vi "ChangePassword.vi"(3 "error in (no error)":errorcluster, 5 "连接模式":enum16{"单机", "联网"}(ring)) -> (0 "error out":errorcluster)   [LabVIEW 2017]
uses:
  <vilib>/Utility/error.llb/DialogType.ctl
  <vilib>/addons/database/Connection.llb/DB Tools Open Connec (String).vi
  <vilib>/addons/database/Connection.llb/Conn Execute.vi
  <vilib>/addons/database/Recordset.llb/Rec Destroy - Connection.vi
  <vilib>/addons/database/NI_Database_API.lvlib
panel:
  in  "取消":bool
  in  "确定":bool
  in  "显示密码":bool
  in  "重复新密码":string
  in  "新   密   码":string
  in  "原   密   码":string
  in  "用   户   名":string(combo)
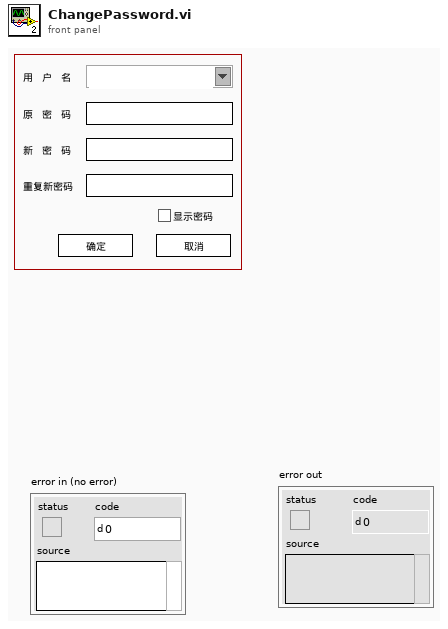
[diagram p1: front panel]
types:
  T1 = typedef "DialogType.ctl" = u16
  T2 = typedef "NI_Database_API.lvlib/Conn ObjectReference.ctl" = refnum<k1>
  T3 = typedef "NI_Database_API.lvlib/Rec ObjectReference.ctl" = refnum<k1>
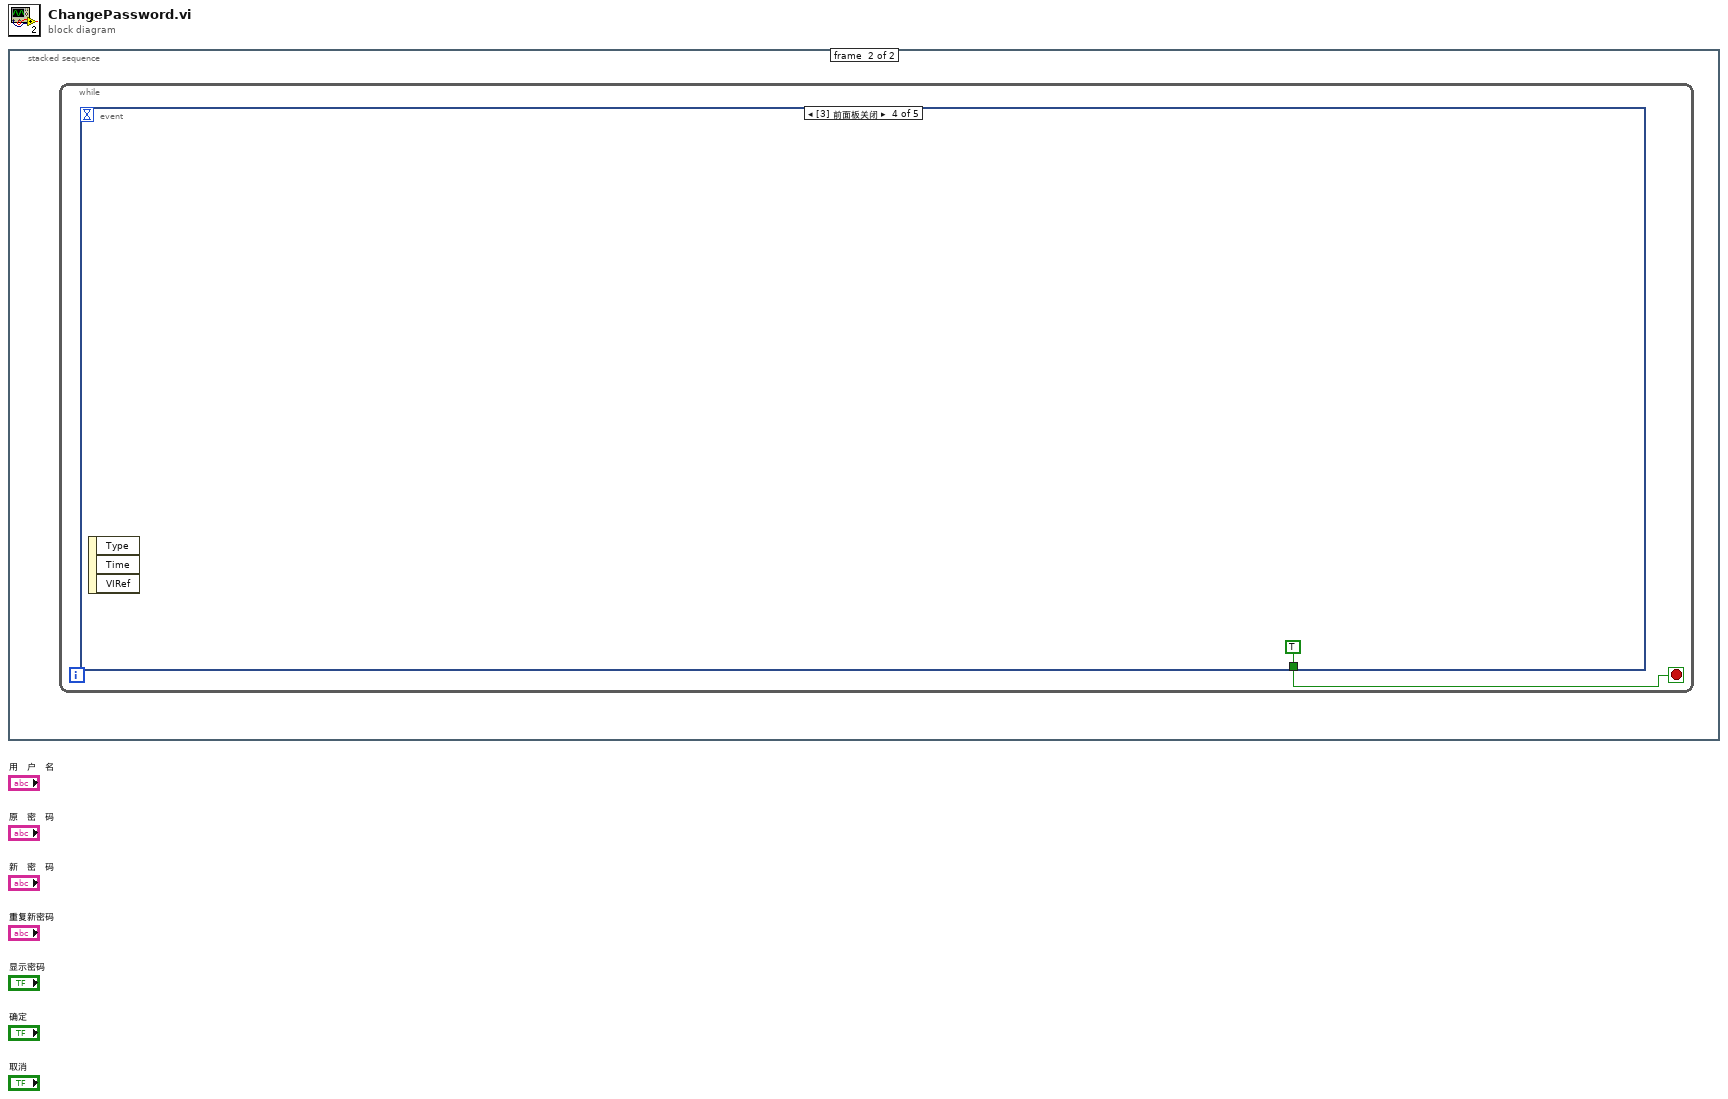
[diagram p0: block diagram]
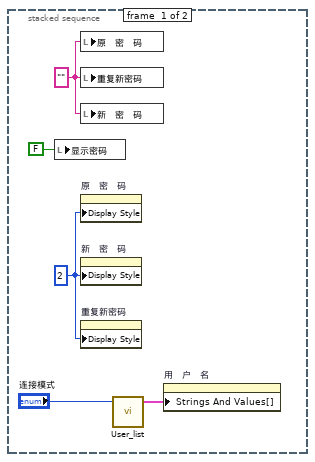
[diagram p2: hidden frame]
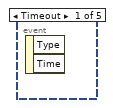
[diagram p3: hidden frame]
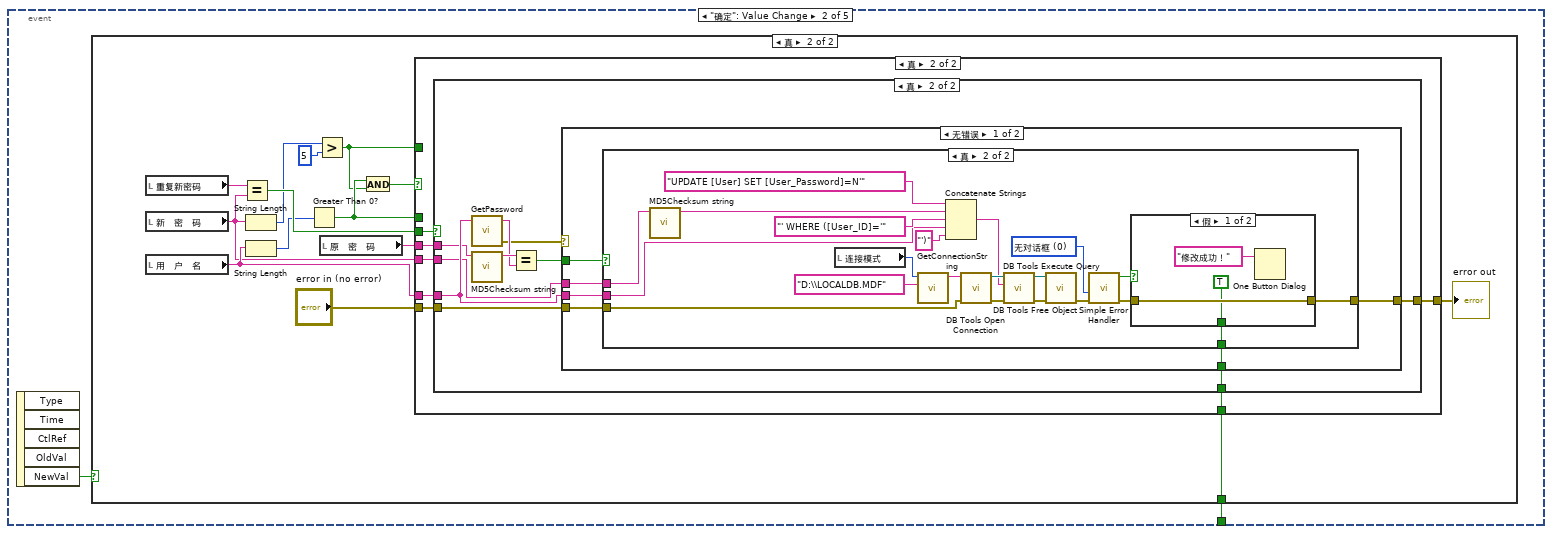
[diagram p4: hidden frame]
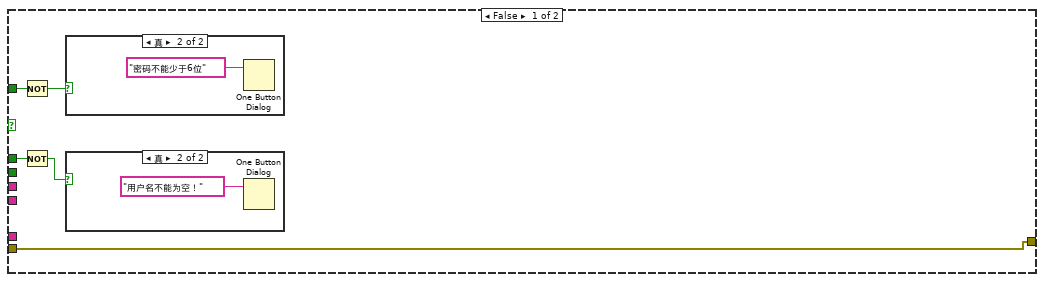
[diagram p6: hidden frame]
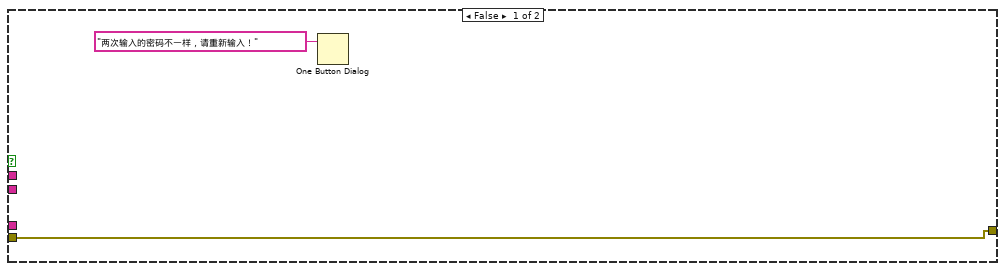
[diagram p9: hidden frame]
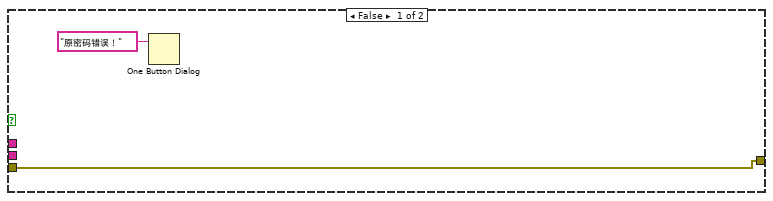
[diagram p10: hidden frame]
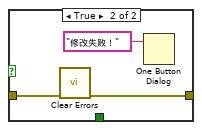
[diagram p11: hidden frame]
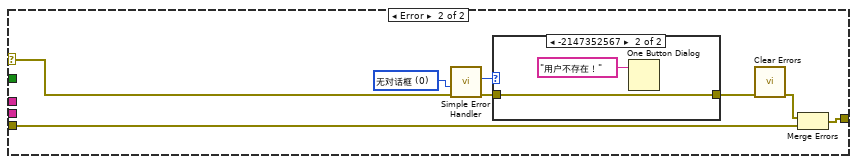
[diagram p12: hidden frame]
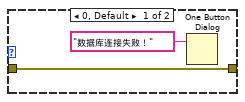
[diagram p13: hidden frame]
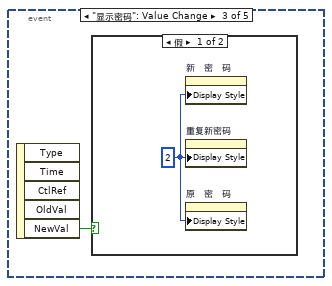
[diagram p14: hidden frame]
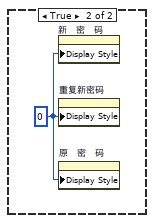
[diagram p15: hidden frame]
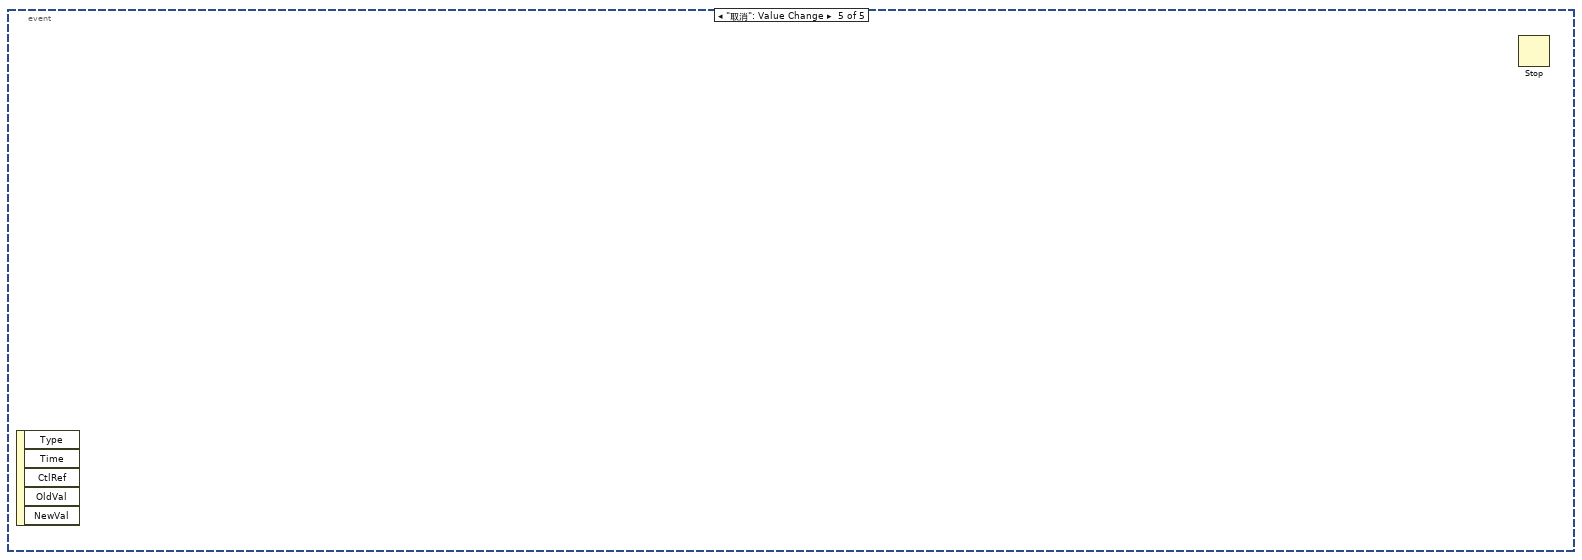
[diagram p16: hidden frame]
diagram:
  n1 = stacked-sequence {
    frame #0 {
      w3 = ""
      w5 = u32 2 ("显示样式")
      n2 = local write "显示密码"(FALSE ("显示密码")) -> ()
      n3 = local write "原   密   码"(w3) -> ()
      n4 = local write "重复新密码"(w3) -> ()
      n5 = local write "新   密   码"(w3) -> ()
      n6 = property on="原   密   码" class="Str"("Display Style"=w5) -> ()  [unwired: 2 in, 2 out]
      n7 = property on="新   密   码" class="Str"("Display Style"=w5) -> ()  [unwired: 2 in, 2 out]
      n8 = property on="重复新密码" class="Str"("Display Style"=w5) -> ()  [unwired: 2 in, 2 out]
      n9 = call "User_list.vi"("连接模式"="连接模式") -> ("User_list"=w2:cluster{string, string}[])  [unwired: 3 in, 1 out]
      n10 = property on="用   户   名" class="CmbBox"("Strings And Values[]"=w2) -> ()  [unwired: 2 in, 2 out]
    }
    frame #1 {
      n11 = while {
        stop <- w6 stop-if-true
        n12 = event shown="[3] 前面板关闭" {
          selector: _ -> [_ _ _ _ _]
          dyn-events: _ -> [_ _ _ _ _]
          timeout: _ -> [_ _ _ _ _]
          tunnel: [_ w7 _ TRUE _] -> w6
          event Timeout {
            n13 = event-data() -> ()  [unwired: 1 in, 2 out]
          }
          event "确定": Value Change {
            n14 = event-data() -> ("NewVal"=w8:bool)  [unwired: 1 in, 4 out]
            n15 = case shown="真" w8 {
              tunnel: [_ w9] -> w7
              frame False {
              }
              frame True {
                n16 = local read "重复新密码"() -> (w20:string)
                n17 = local read "新   密   码"() -> (w13:string)
                n18 = local read "用   户   名"() -> (w16:string)
                n19 = Equal?(x=w20, y=w13) -> (x = y?=w21:bool)
                n20 = String Length(string=w13) -> (length=w15:i32)
                n21 = String Length(string=w16) -> (length=w17:i32)
                n22 = Greater Than 0?(x=w17) -> (x > 0?=w11:bool)
                n23 = Greater?(x=w15, y=5) -> (0:w10:bool)
                n24 = local read "原   密   码"() -> (w22:string)
                n25 = And(x=w11, y=w10) -> (x .and. y?=w12:bool)
                n26 = case shown="真" w12 {
                  tunnel: w13 -> [_ w36]
                  tunnel: w22 -> [_ w35]
                  tunnel: w16 -> [_ w34]
                  tunnel: w21 -> [_ w33]
                  tunnel: [w27 w32] -> w19
                  tunnel: "error in (no error)" -> [w27 w31]
                  tunnel: w11 -> [w26 _]
                  tunnel: w10 -> [w24 _]
                  tunnel: [_ w30] -> w9
                  frame False {
                    n27 = Not(x=w24) -> (.not. x?=w23:bool)
                    n28 = Not(x=w26) -> (.not. x?=w25:bool)
                    n29 = case shown="真" w23 {
                      frame False {
                      }
                      frame True {
                        n30 = One Button Dialog(message="密码不能少于6位" ("消息")) -> ()  [unwired: 1 in, 1 out]
                      }
                    }
                    n31 = case shown="真" w25 {
                      frame False {
                      }
                      frame True {
                        n32 = One Button Dialog(message="用户名不能为空！" ("消息")) -> ()  [unwired: 1 in, 1 out]
                      }
                    }
                  }
                  frame True {
                    n33 = case shown="真" w33 {
                      tunnel: w31 -> [w38 w48]
                      tunnel: [w38 w47] -> w32
                      tunnel: w34 -> [_ w44]
                      tunnel: w35 -> [_ w43]
                      tunnel: w36 -> [_ w42]
                      tunnel: [_ w39] -> w30
                      frame False {
                        n34 = One Button Dialog(message="两次输入的密码不一样，请重新输入！" ("消息")) -> ()  [unwired: 1 in, 1 out]
                      }
                      frame True {
                        n35 = call "GetPassword.vi"("User_Name"=w44) -> ("error out"=w40:errorcluster, "Password"=w45:string)  [unwired: 2 in, 1 out]
                        n36 = call <vilib>:"MD5Checksum string.vi"("Message String"=w43) -> ("MD5 message-digest"=w46:string)  [unwired: 10 in]
                        n37 = Equal?(x=w46, y=w45) -> (x = y?=w41:bool)
                        n38 = case shown="无错误" w40 {
                          selector: w40 -> [_ w91]
                          tunnel: w48 -> [w54 w90]
                          tunnel: [w53 w89] -> w47
                          tunnel: w44 -> [w52 _]
                          tunnel: w42 -> [w51 _]
                          tunnel: w41 -> [w50 _]
                          tunnel: [w49 _] -> w39
                          frame No Error {
                            n39 = case shown="真" w50 {
                              tunnel: w54 -> [w56 w71]
                              tunnel: [w56 w68] -> w53
                              tunnel: w51 -> [_ w59]
                              tunnel: w52 -> [_ w60]
                              tunnel: [_ w57] -> w49
                              frame False {
                                n40 = One Button Dialog(message="原密码错误！" ("消息")) -> ()  [unwired: 1 in, 1 out]
                              }
                              frame True {
                                w72 = T1 0 items=["无对话框", "确定信息", "继续或停止信息", "确定信息＋警告", "继续/停止+警告"] ("type of dialog (OK msg:1)")
                                n41 = call <vilib>:"MD5Checksum string.vi"("Message String"=w59) -> ("MD5 message-digest"=w58:string)  [unwired: 10 in]
                                n42 = local read "连接模式"() -> (w61:enum16{"单机", "联网"})
                                n43 = call "GetConnectionString.vi"("Database Name"="D:\\LOCALDB.MDF", "连接模式"=w61) -> ("连接字符串"=w63:string)  [unwired: 4 in, 1 out]
                                n44 = Concatenate Strings("UPDATE [User] SET [User_Password]=N'", w58, "' WHERE ([User_ID]='", w60, "')") -> (w64:string)
                                n45 = call-poly <vilib>:"DB Tools Open Connection.vi"("error in (no error)"=w71, "connection information"=w63) -> ("error out"=w77:errorcluster, "connection reference"=w76:T2)  [unwired: 6 in]
                                n46 = call-poly <vilib>:"DB Tools Execute Query.vi"("error in (no error)"=w77, "SQL query"=w64, "connection reference"=w76) -> ("error out"=w75:errorcluster, "recordset reference"=w74:T3)  [unwired: 5 in]
                                n47 = call-poly <vilib>:"DB Tools Free Object.vi"("error in (no error)"=w75, "recordset reference"=w74) -> ("error out"=w73:errorcluster)  [unwired: 8 in, 1 out]
                                n48 = call <vilib>:"Simple Error Handler.vi"("type of dialog (OK msg:1)"=w72, "error in (no error)"=w73) -> ("error?"=w70:bool, "error out"=w69:errorcluster)  [unwired: 3 in, 3 out]
                                n49 = case shown="假" w70 {
                                tunnel: w69 -> [w79 w81]
                                tunnel: [w79 w82] -> w68
                                tunnel: [TRUE _] -> w57
                                frame False {
                                n50 = One Button Dialog(message="修改成功！" ("消息")) -> ()  [unwired: 1 in, 1 out]
                                }
                                frame True {
                                n51 = call <vilib>:"Clear Errors.vi"("error in (no error)"=w81) -> ("error out"=w82:errorcluster)  [unwired: 5 in, 1 out]
                                n52 = One Button Dialog(message="修改失败！" ("消息")) -> ()  [unwired: 1 in, 1 out]
                                }
                                }
                              }
                            }
                          }
                          frame Error {
                            w88 = T1 0 items=["无对话框", "确定信息", "继续或停止信息", "确定信息＋警告", "继续/停止+警告"] ("type of dialog (OK msg:1)")
                            n53 = call <vilib>:"Simple Error Handler.vi"("type of dialog (OK msg:1)"=w88, "error in (no error)"=w91) -> ("code out"=w87:i32, "error out"=w86:errorcluster)  [unwired: 3 in, 3 out]
                            n54 = case shown="-2147352567" w87 {
                              tunnel: w86 -> [w92 w94]
                              tunnel: [w92 w94] -> w85
                              frame 0, Default {
                                n55 = One Button Dialog(message="数据库连接失败！" ("消息")) -> ()  [unwired: 1 in, 1 out]
                              }
                              frame -2147352567 {
                                n56 = One Button Dialog(message="用户不存在！" ("消息")) -> ()  [unwired: 1 in, 1 out]
                              }
                            }
                            n57 = call <vilib>:"Clear Errors.vi"("error in (no error)"=w85) -> ("error out"=w84:errorcluster)  [unwired: 5 in, 1 out]
                            n58 = Merge Errors(w84, w90) -> (w89:errorcluster)
                          }
                        }
                      }
                    }
                  }
                }
                "error out" <- w19
              }
            }
          }
          event "显示密码": Value Change {
            n59 = event-data() -> ("NewVal"=w96:bool)  [unwired: 1 in, 4 out]
            n60 = case shown="假" w96 {
              frame False {
                w97 = u32 2 ("显示样式")
                n61 = property on="新   密   码" class="Str"("Display Style"=w97) -> ()  [unwired: 2 in, 2 out]
                n62 = property on="重复新密码" class="Str"("Display Style"=w97) -> ()  [unwired: 2 in, 2 out]
                n63 = property on="原   密   码" class="Str"("Display Style"=w97) -> ()  [unwired: 2 in, 2 out]
              }
              frame True {
                w98 = u32 0 ("显示样式")
                n64 = property on="新   密   码" class="Str"("Display Style"=w98) -> ()  [unwired: 2 in, 2 out]
                n65 = property on="重复新密码" class="Str"("Display Style"=w98) -> ()  [unwired: 2 in, 2 out]
                n66 = property on="原   密   码" class="Str"("Display Style"=w98) -> ()  [unwired: 2 in, 2 out]
              }
            }
          }
          event Panel Close {
            n67 = event-data() -> ()  [unwired: 1 in, 3 out]
          }
          event "取消": Value Change {
            n68 = event-data() -> ()  [unwired: 1 in, 5 out]
            n69 = Stop() -> ()  [unwired: 1 in]
          }
        }
      }
    }
  }
